vi "Drag & Drop New Single.vi"(0 "Reference In":refnum<vi>, 3 "error in":errorcluster) -> (7 "References out":T1, 10 "error out":errorcluster)   [LabVIEW 2015]
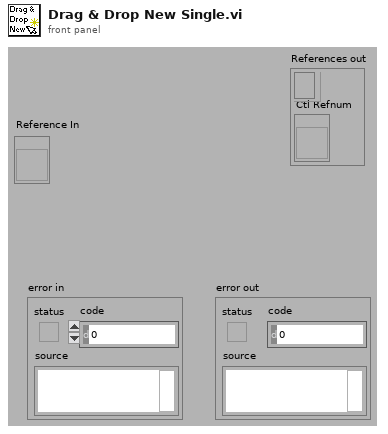
[diagram p1: front panel]
types:
  T1 = cluster{"Event Registration Refnum":refnum<event-registration>, "Ctl Refnum":refnum<vi>}
  T2 = cluster{"Event Registration Refnum":refnum<event-registration>, "Reference In":refnum<vi>}
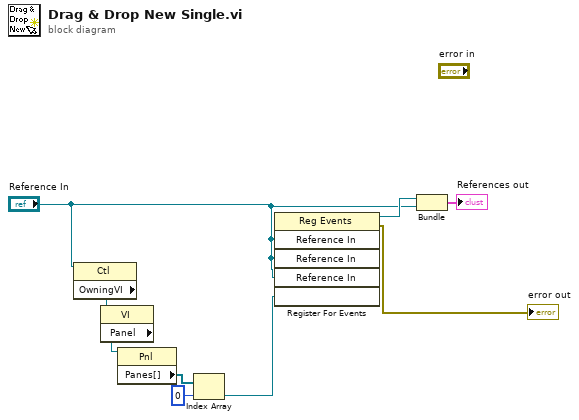
[diagram p0: block diagram]
diagram:
  n1 = property class="Ctl"(reference="Reference In") -> ("OwningVI"=w7:refnum<vi>)  [unwired: 1 in, 2 out]
  n2 = property class="VI"(reference=w7) -> ("Panel"=w6:refnum<vi>)  [unwired: 1 in, 2 out]
  n3 = property class="Pnl"(reference=w6) -> ("Panes[]"=w5:refnum<vi>[])  [unwired: 1 in, 2 out]
  n4 = Index Array(array=w5, index=0) -> (element=w3:refnum<vi>)
  n5 = register-events("Reference In", "Reference In", "Reference In", w3) -> (reference out=w8:refnum<event-registration>, error out=→"error out":errorcluster)  [unwired: 2 in]
  n6 = Bundle("Event Registration Refnum"=w8, "Reference In"="Reference In") -> (→"References out":T2)  [unwired: 1 out]
